vi "String Length, Concatenate , String Subset Part1.vi"() -> ()   [LabVIEW 2020]
panel:
  out "substring":string
  out "concatenated string":string
  out "length":i32
  in  "String":string
  # "Part 1"
  # "String Length, Concatenate Strings, String Subset"
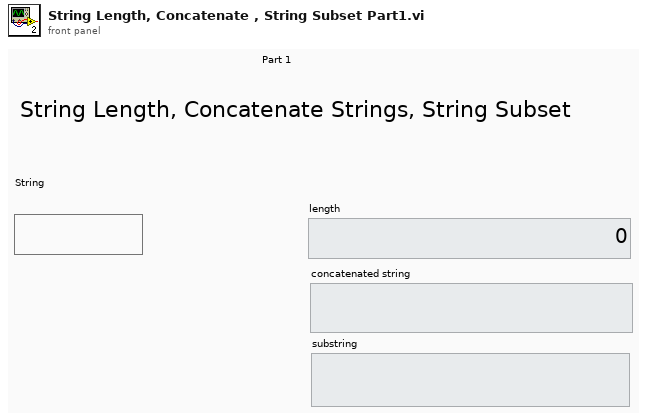
[diagram p1: front panel]
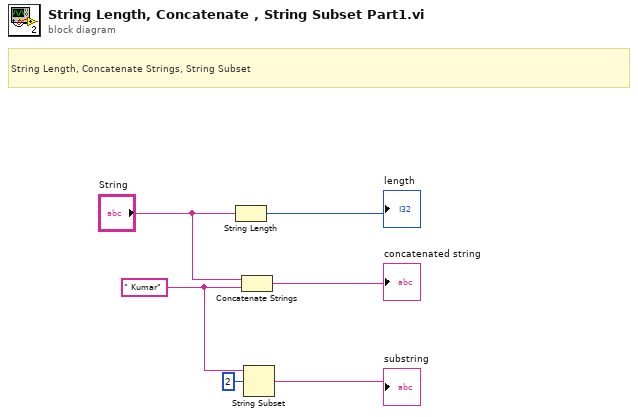
[diagram p0: block diagram]
diagram:
  w3 = " Kumar" ("string")
  # "String Length, Concatenate Strings, String Subset"
  n1 = String Length(string="String") -> (length=→"length":i32)
  n2 = Concatenate Strings "Concatenate Strings"("String", w3) -> (→"concatenated string":string)
  n3 = String Subset(string=w3, offset (0)=2) -> (substring=→"substring":string)  [unwired: 1 in]
